vi "Recieve Acknowledge Initialized.vi"(8 "error in (no error)":errorcluster, 9 "Requestor":string, 10 "Requestee":string, 11 "Mag Lab Measure Controller in":refnum<class "Mag Lab Measure Controller.lvclass">) -> (0 "error out":errorcluster, 3 "Mag Lab Measure Controller out":refnum<class "Mag Lab Measure Controller.lvclass">)   [LabVIEW 2015, in "Mag Lab Measure Controller.lvclass"]
uses:
  Mag Lab Measure Controller.lvclass
  Mag Lab Root/Mag Lab Root.lvclass/Mag Lab Root.ctl
  Mag Lab Root Messages/Recieve Acknowledge Initialized Msg/Recieve Acknowledge Initialized Msg.lvclass/Recieve Acknowledge Initialized Msg.ctl
  <vilib>/ActorFramework/Message Enqueuer/Message Enqueuer.lvclass/Message Enqueuer.ctl
  Mag Lab Measure Controller.lvclass/Mag Lab Measure Controller.ctl
  <vilib>/ActorFramework/Message Enqueuer/Enqueue.vi
  <vilib>/ActorFramework/Message Priority Queue/Priority Enqueue.vi
  Mag Lab Root Messages/Recieve Acknowledge Initialized Msg/Recieve Acknowledge Initialized Msg.lvclass
  Compound Measurement/Compound Measurement.lvclass
  Mag Lab Measure Base/Mag Lab Measure Base.lvclass
  Mag Lab Root/Mag Lab Root.lvclass
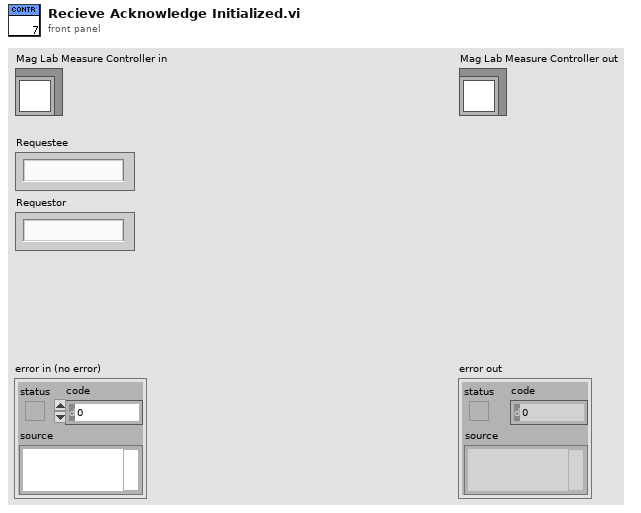
[diagram p1: front panel]
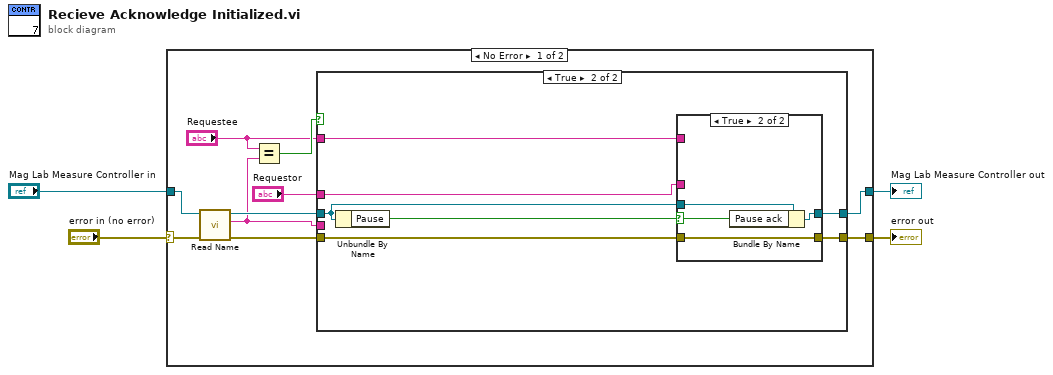
[diagram p0: block diagram]
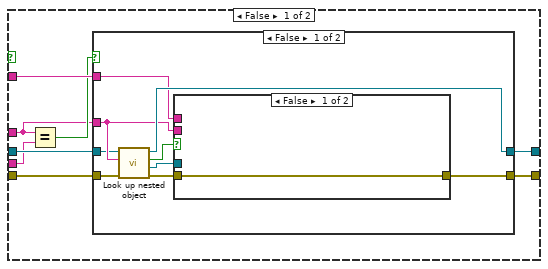
[diagram p2: hidden frame]
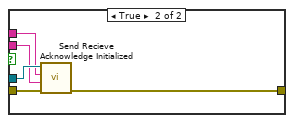
[diagram p3: hidden frame]
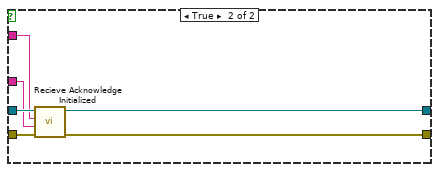
[diagram p4: hidden frame]
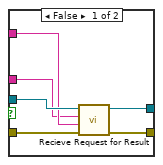
[diagram p5: hidden frame]
diagram:
  n1 = case shown="No Error" "error in (no error)" {
    selector: "error in (no error)" -> [w11 w62]
    tunnel: [w14 w62] -> w3
    tunnel: [w13 w61] -> w1
    tunnel: "Mag Lab Measure Controller in" -> [w12 w61]
    frame No Error {
      n2 = call "Read Name.vi"("error in (no error)"=w11, "Mag Lab Root in"=w12) -> ("error out"=w9:errorcluster, "Name"=w5:string, "Mag Lab Root out"=w10:refnum<class "Mag Lab Measure Controller.lvclass">)  [unwired: 7 in]
      n3 = Equal?(x="Requestee", y=w5) -> (x = y?=w7:bool)
      n4 = case shown="True" w7 {
        tunnel: [w22 w47] -> w14
        tunnel: [w21 w46] -> w13
        tunnel: "Requestee" -> [w20 w49]
        tunnel: w10 -> [w18 w45]
        tunnel: w9 -> [w17 w50]
        tunnel: "Requestor" -> [w16 w48]
        tunnel: w5 -> [w15 _]
        frame False {
          n5 = Equal?(x=w16, y=w15) -> (x = y?=w19:bool)
          n6 = case shown="False" w19 {
            tunnel: [w29 w39] -> w22
            tunnel: [w28 w38] -> w21
            tunnel: w20 -> [w27 w41]
            tunnel: w16 -> [w25 w40]
            tunnel: w18 -> [w23 w43]
            tunnel: w17 -> [w24 w42]
            frame False {
              n7 = call "Look up nested object.vi"("error in (no error)"=w24, "Object name"=w25, "Mag Lab Measure Base in"=w23) -> ("error out"=w30:errorcluster, "Object Queue"=w31:refnum<class "Message Enqueuer.lvclass">, "Found?"=w26:bool, "Mag Lab Measure Base out"=w28:refnum<class "Mag Lab Measure Controller.lvclass">)  [unwired: 5 in]
              n8 = case shown="False" w26 {
                tunnel: w31 -> [_ w37]
                tunnel: w30 -> [w32 w36]
                tunnel: [w32 w35] -> w29
                tunnel: w25 -> [_ w34]
                tunnel: w27 -> [_ w33]
                frame False {
                }
                frame True {
                  n9 = call "Send Recieve Acknowledge Initialized.vi"("error in (no error)"=w36, "Requestor"=w34, "Requestee"=w33, "Message Enqueuer"=w37) -> ("error out"=w35:errorcluster)  [unwired: 6 in, 1 out]
                }
              }
            }
            frame True {
              n10 = call-parent "Recieve Acknowledge Initialized.vi"("error in (no error)"=w42, "Requestor"=w40, "Requestee"=w41, "Compound Measurement in"=w43) -> ("error out"=w39:errorcluster, "Compound Measurement out"=w38:refnum<class "Mag Lab Measure Controller.lvclass">)  [unwired: 6 in]
            }
          }
        }
        frame True {
          n11 = Unbundle By Name(w45) -> ("Pause"=w44:bool)
          n12 = case shown="True" w44 {
            selector: w44 -> [_ w59]
            tunnel: w45 -> [w56 w60]
            tunnel: w50 -> [w55 w58]
            tunnel: w49 -> [w54 _]
            tunnel: w48 -> [w53 _]
            tunnel: [w52 w58] -> w47
            tunnel: [w51 w57] -> w46
            frame False {
              n13 = call-dynamic "Recieve Request for Result.vi"("error in (no error)"=w55, "Requestor"=w54, "Requestee"=w53, "Mag Lab Measure Controller in"=w56) -> ("error out"=w52:errorcluster, "Mag Lab Measure Controller out"=w51:refnum<class "Mag Lab Measure Controller.lvclass">)  [unwired: 6 in]
            }
            frame True {
              n14 = Bundle By Name(cluster=w60, "Pause ack"=w59) -> (w57:refnum<class "Mag Lab Measure Controller.lvclass">)
            }
          }
        }
      }
    }
    frame Error {
    }
  }
  "error out" <- w3
  "Mag Lab Measure Controller out" <- w1
